vi "Powerboard_Controller Test.vi"() -> ()   [LabVIEW 2018]
uses:
  LVU examples/SubVIs/Global textParse.vi
  <instrlib>/RIGOL DS1000 Series/RIGOL DS1000 Series.lvlib
  <vilib>/measure/NI_MAPro.lvlib
  <vilib>/measure/mascope.llb/Amplitude and Levels 1 chan.vi
  <vilib>/Utility/file.llb/Read Delimited Spreadsheet (string).vi
panel:
  out "Y min 2":dbl format="%0.2f"
  out "Y max 2":dbl format="%0.2f"
  out "Y min":dbl format="%0.2f"
  out "Y max":dbl format="%0.2f"
  out "Digital Display 2":dbl
  out "Boolean 3":bool
  out "Boolean 2":bool
  out "Boolean":bool
  out "Out 5":dbl
  out "Out 4":dbl
  out "Out 3":dbl
  out "Out 2":dbl
  out "Out 1":dbl
  in  "Tab Control":T1(tab)
  in  "Department":string
  in  "Operator Name":string="ID-0"
  in  "SpecSheet Scan":string
  out "Good":bool
  in  "E-STOP":bool
  out "Bad":bool
  out "File Path":string
  out "File Name":string
  in  "Department":bool
  in  "Name":bool
  out "Boolean 4":bool
  out "Boolean 5":bool
  in  "Barcode Scan":string
  in  "VISA Waveform Generator":refnum<visa-resource-name>
  in  "VISA MultiMeter":refnum<visa-resource-name>
  in  "VISA Oscilloscope":refnum<visa-resource-name>
  out "Vmicr0":bool
  out "Vfet Driver":bool
  out "Primary":dbl(slide) caption="Secondary" scale=0.0..3000.0
  in  "Serial Port":refnum<visa-resource-name>
  out "I limit":bool
  out "I Limit":string
  out "Firmware 2":bool
  out "Firmware":string
  out "IRcomp 2":bool
  out "IRcomp":string
  out "DG":bool
  out "DM":bool
  out "DS":bool
  out "bar code read":string
  in  "stop":bool
  in  "bar code":string
  out "concatenated string":string
  out "error?":bool
  in  "Documentation":u16(ring) items=["SW Version", "Powerboard_Controller", "Equipment Test"]
  out "SW Version":string[][](array[string])
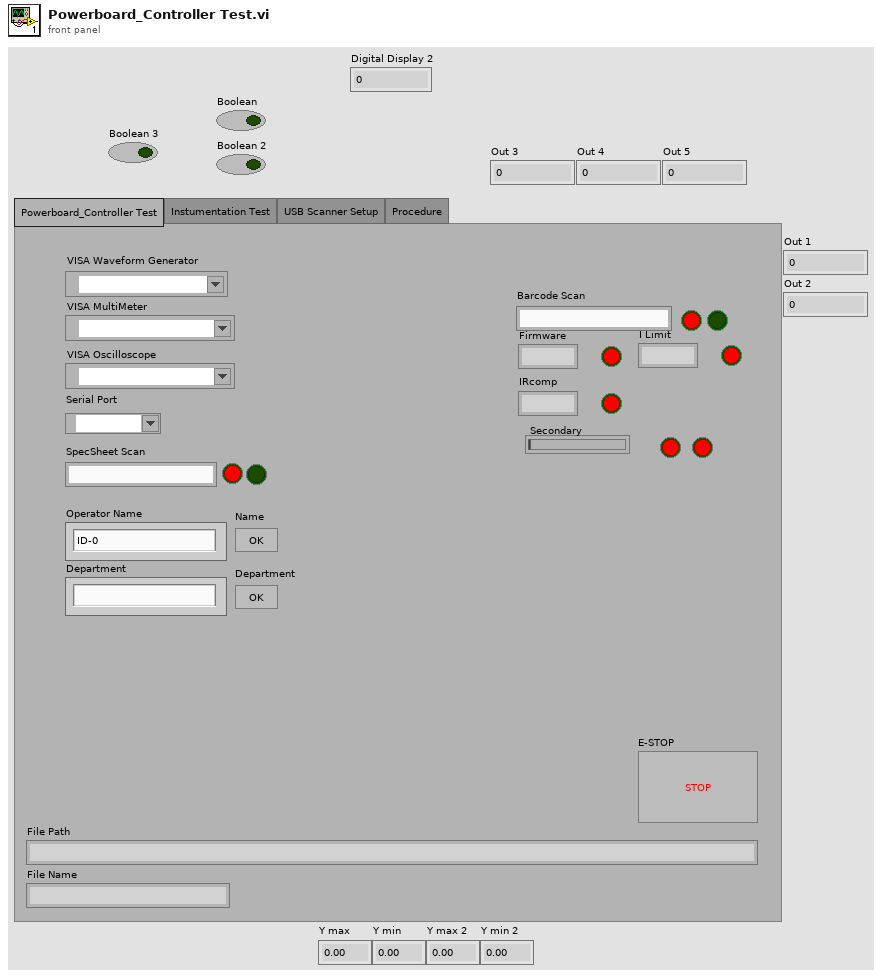
[diagram p1: front panel]
types:
  T1 = enum32{"Powerboard_Controller Test", "Instumentation Test", "USB Scanner Setup", "Procedure"}
  T2 = enum16{"Always On", "Always Off", "Off While Running"}
  T3 = enum16{"Initialize", "SW Read", "Secondary", "Incline", "Primary", "Motor", "Another", "Fail", "Close"}
  T4 = enum16{"Console unloaded", "Console loaded", "pass through", "fail"}
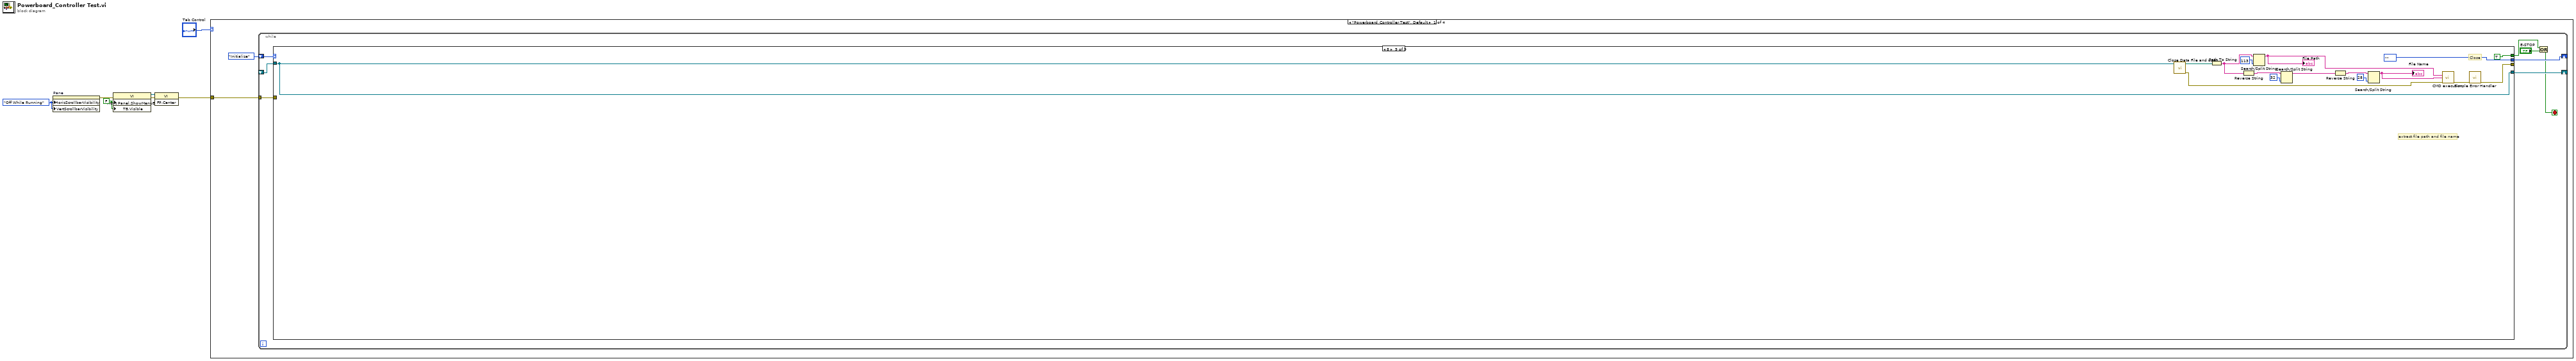
[diagram p0: block diagram]
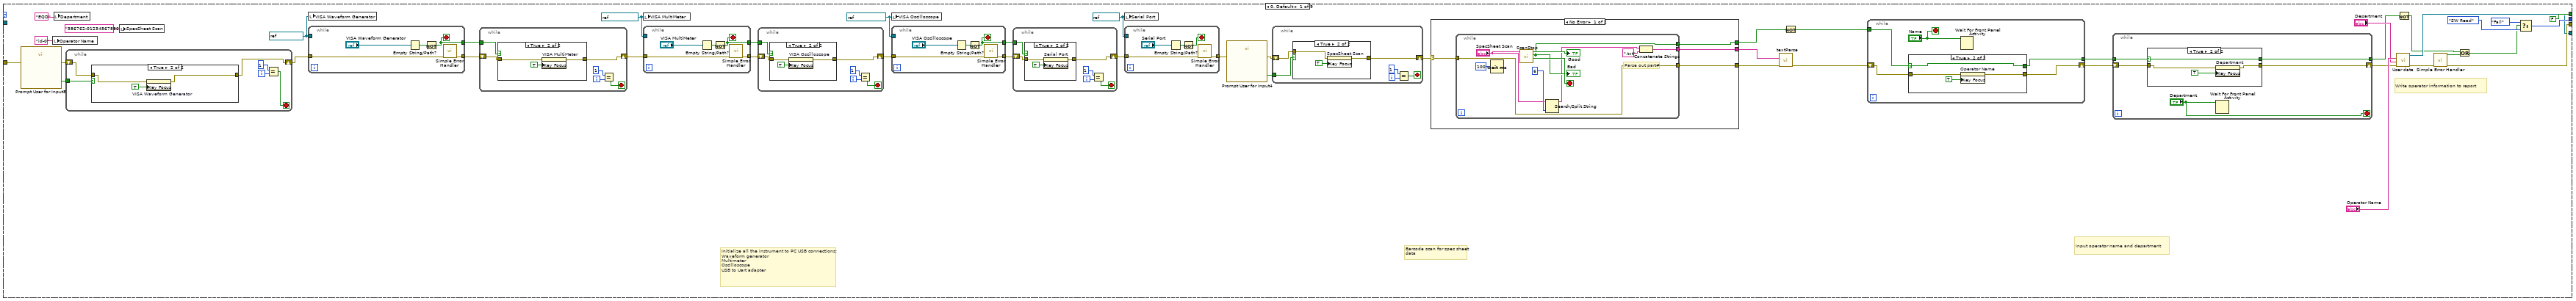
[diagram p2: hidden frame]
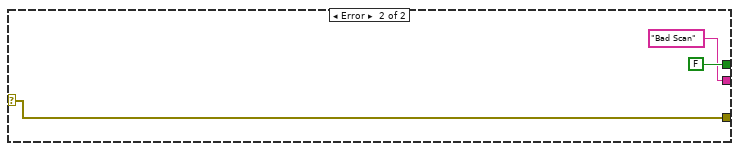
[diagram p10: hidden frame]
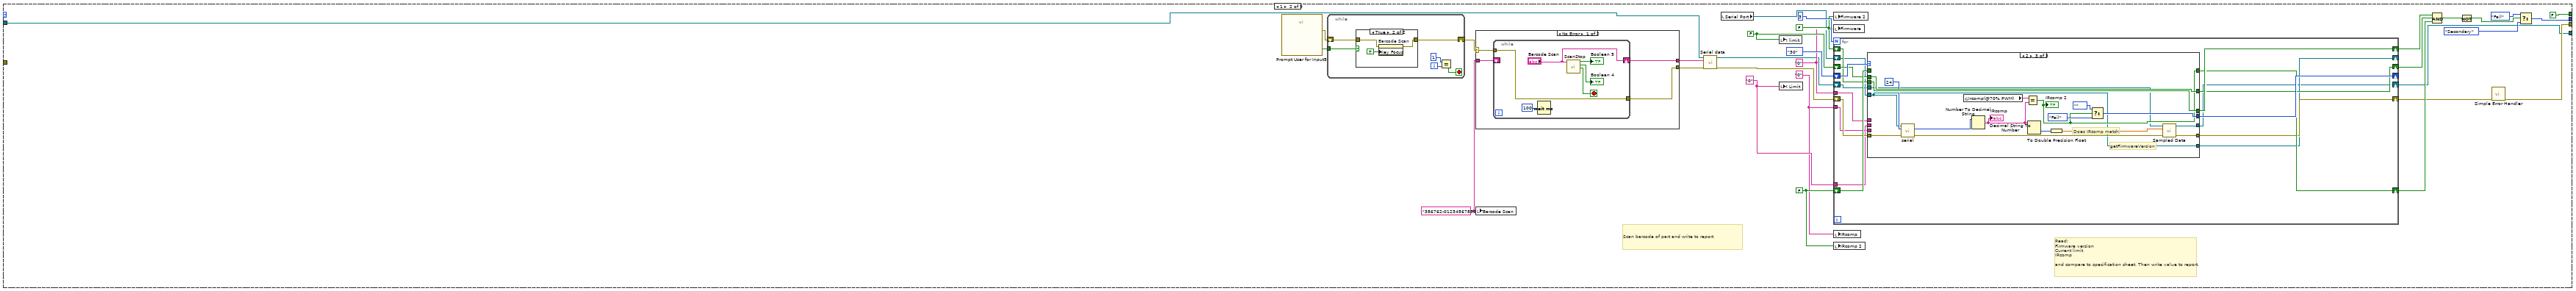
[diagram p11: hidden frame]
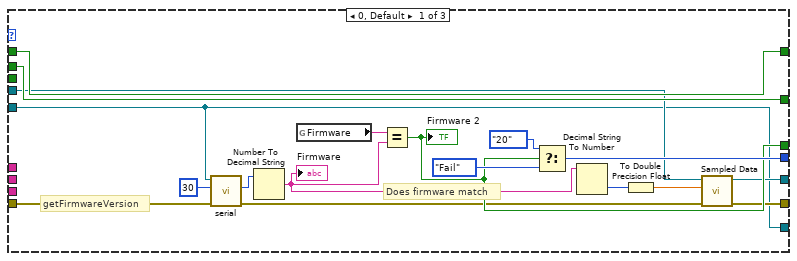
[diagram p12: hidden frame]
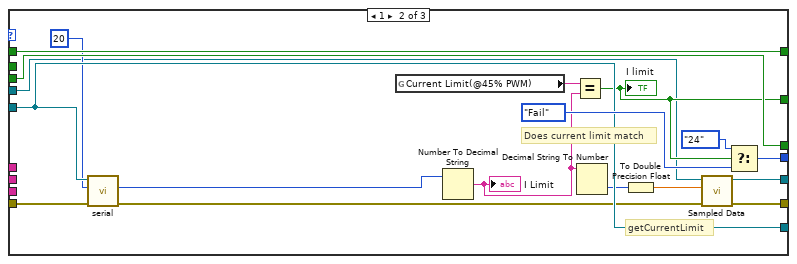
[diagram p13: hidden frame]
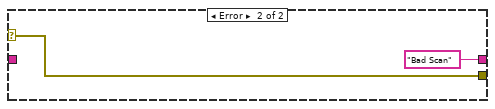
[diagram p15: hidden frame]
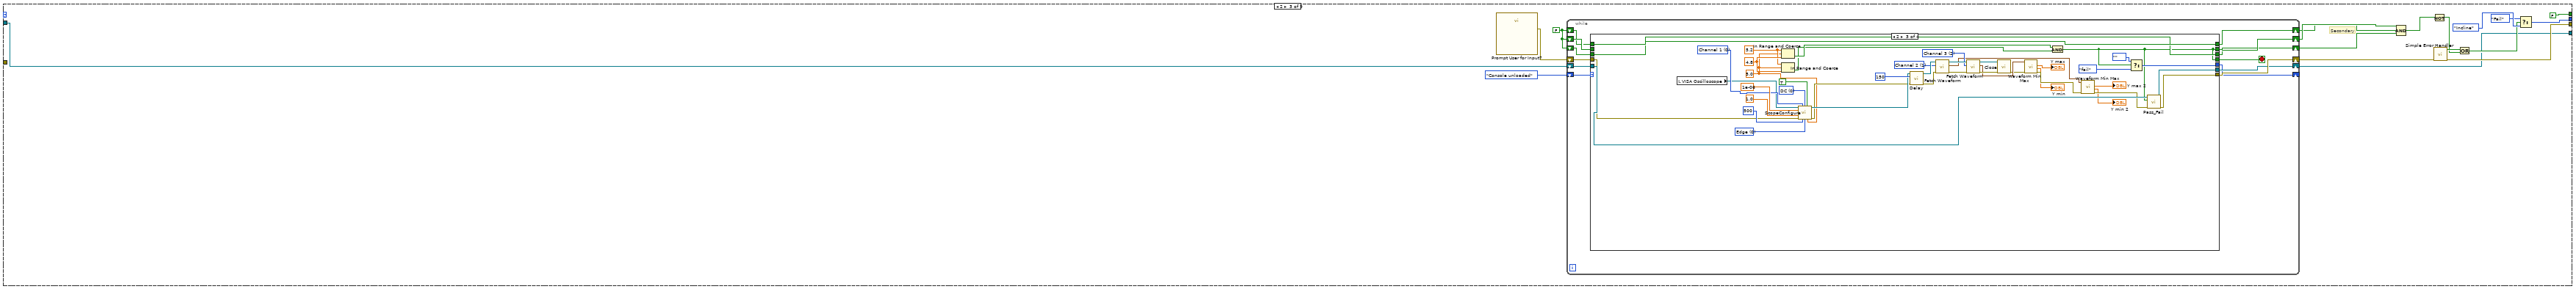
[diagram p16: hidden frame]
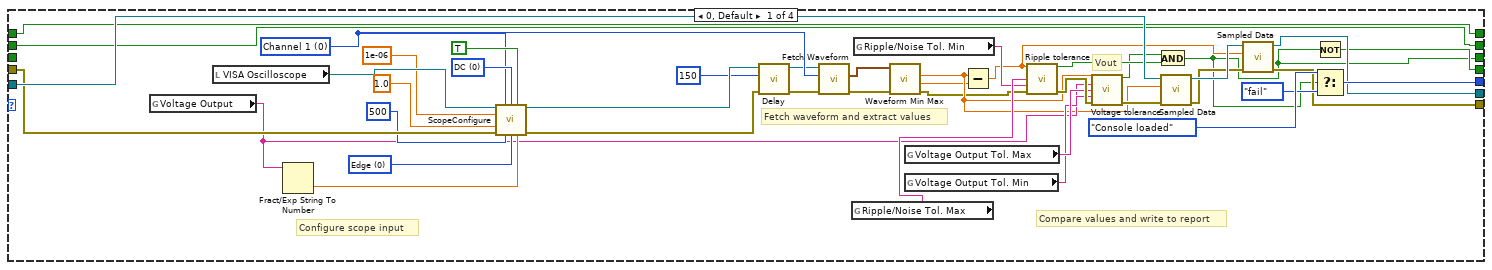
[diagram p17: hidden frame]
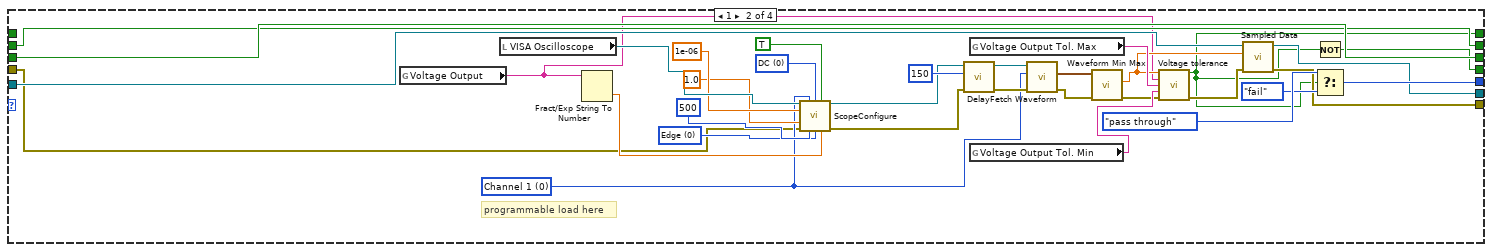
[diagram p18: hidden frame]
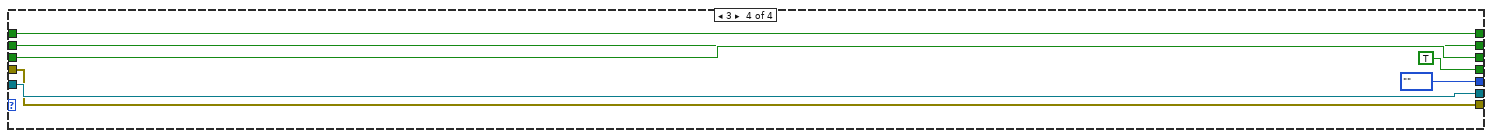
[diagram p19: hidden frame]
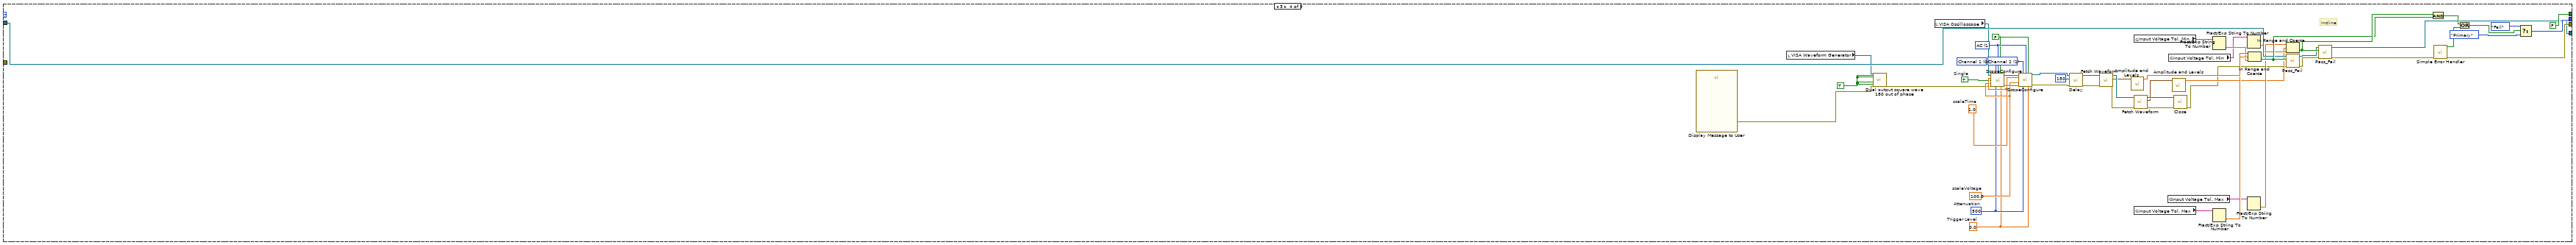
[diagram p20: hidden frame]
diagram:
  w3 = FALSE ("Front Panel Window:Show Menu Bar")
  w2 = T2."Off While Running" ("Vertical Scrollbar Visibility")
  n1 = property on="Pane" class="Pane"("HorizScrollbarVisibility"=w2, "VertScrollbarVisibility"=w2) -> (error out=w4:errorcluster)  [unwired: 2 in, 1 out]
  n2 = property class="VI"(error in=w4, "Front Panel.ShowMenuBar"=w3, "TB.Visible"=w3) -> (reference out=w6:refnum<vi>, error out=w5:errorcluster)  [unwired: 1 in]
  n3 = invoke class="VI" method="FP.Center"(reference=w6, error in=w5) -> (error out=w1:errorcluster)  [unwired: 1 in, 2 out]
  n4 = case shown="\"Powerboard_Controller Test\", Default" "Tab Control" {
    tunnel: w1 -> [w8 _ _ _]
    frame "Powerboard_Controller Test", Default {
      n5 = while {
        shift-right: [w17] -> _
        shift-left: T3."Initialize" -> [w16]
        shift-right: [w15] -> _
        shift-left: _ -> [w14]
        tunnel: w8 -> [w10]
        stop <- w11 stop-if-true
        n6 = case shown="8" w16 {
          tunnel: [w62 w200 w309 w501 w532 w583 w597 T3."Another" enum16{""}.""] -> w17
          tunnel: [w61 w201 w310 w500 w531 w584 w596 w605 w621] -> _
          tunnel: [w50 w174 w303 w491 w527 w580 w595 w603 w619] -> w15
          tunnel: w14 -> [_ w190 w304 w493 w529 w578 w595 w602 w619]
          tunnel: [FALSE ("error?") FALSE ("error?") FALSE ("error?") FALSE ("error?") FALSE ("error?") FALSE ("error?") FALSE ("error?") w604 TRUE ("error?")] -> w12
          tunnel: w10 -> [w22 _ _ _ _ _ _ _ _]
          frame 0, Default {
            w26 = refnum<visa-resource-name> "COM4" ("VISA MultiMeter")
            w25 = refnum<visa-resource-name> "DemoScope" ("VISA MultiMeter")
            w24 = refnum<visa-resource-name> "Multimeter" ("VISA MultiMeter")
            w23 = refnum<visa-resource-name> "Generator" ("VISA Waveform Generator")
            # "Write operator information to report"
            # "Input operator name and department"
            # "Barcode scan for spec sheet data"
            # "Initialize all the instrument to PC USB connections:\nWaveform generator\nMultimeter\nOscilloscope\nUSB to Uart adapter"
            n7 = call "Prompt User for Input8"("error in (no error)"=w22) -> ("OK"=w28:bool, "error out"=w27:errorcluster)  [unwired: 17 in]
            n8 = local write "Operator Name"("id-0") -> ()
            n9 = local write "Department"("EQD") -> ()
            n10 = while {
              tunnel: w28 -> [w116]
              shift-right: [w118] -> w29
              shift-left: w27 -> [w117]
              i -> [w115]
              stop <- w113 stop-if-true
              n11 = case shown="True" w116 {
                tunnel: [w119 w122] -> w118
                tunnel: w117 -> [w119 w121]
                frame False {
                }
                frame True {
                  n12 = property on="VISA Waveform Generator" class="VISAName"(error in=w121, "Key Focus"=TRUE) -> (error out=w122:errorcluster)  [unwired: 1 in, 1 out]
                }
              }
              n13 = Equal?(x=1, y=w115) -> (x = y?=w113:bool)
            }
            n14 = local write "SpecSheet Scan"("386762-01234567890") -> ()
            n15 = local write "VISA Waveform Generator"(w23) -> ()
            n16 = while {
              tunnel: w29 -> [w112]
              tunnel: [w111] -> w30
              tunnel: w23 -> [_]
              tunnel: [w108] -> w31
              stop <- w108 stop-if-true
              n17 = Empty String/Path?(string/path="VISA Waveform Generator") -> (empty?=w109:bool)
              n18 = Not(x=w109) -> (.not. x?=w108:bool)
              n19 = call <vilib>:"Simple Error Handler.vi"("error in (no error)"=w112) -> ("error out"=w111:errorcluster)  [unwired: 4 in, 4 out]
            }
            n20 = while {
              tunnel: w31 -> [w101]
              shift-right: [w103] -> w32
              shift-left: w30 -> [w102]
              i -> [w100]
              stop <- w98 stop-if-true
              n21 = case shown="True" w101 {
                tunnel: [w104 w107] -> w103
                tunnel: w102 -> [w104 w106]
                frame False {
                }
                frame True {
                  n22 = property on="VISA MultiMeter" class="VISAName"(error in=w106, "Key Focus"=TRUE) -> (error out=w107:errorcluster)  [unwired: 1 in, 1 out]
                }
              }
              n23 = Equal?(x=1, y=w100) -> (x = y?=w98:bool)
            }
            n24 = local write "VISA MultiMeter"(w24) -> ()
            n25 = while {
              tunnel: w32 -> [w97]
              tunnel: [w96] -> w34
              tunnel: [w94] -> w35
              tunnel: w24 -> [_]
              stop <- w94 stop-if-true
              n26 = Empty String/Path?(string/path="VISA MultiMeter") -> (empty?=w95:bool)
              n27 = Not(x=w95) -> (.not. x?=w94:bool)
              n28 = call <vilib>:"Simple Error Handler.vi"("error in (no error)"=w97) -> ("error out"=w96:errorcluster)  [unwired: 4 in, 4 out]
            }
            n29 = while {
              tunnel: w35 -> [w86]
              shift-right: [w88] -> w33
              shift-left: w34 -> [w87]
              i -> [w85]
              stop <- w83 stop-if-true
              n30 = case shown="True" w86 {
                tunnel: [w89 w92] -> w88
                tunnel: w87 -> [w89 w91]
                frame False {
                }
                frame True {
                  n31 = property on="VISA Oscilloscope" class="VISAName"(error in=w91, "Key Focus"=TRUE) -> (error out=w92:errorcluster)  [unwired: 1 in, 1 out]
                }
              }
              n32 = Equal?(x=1, y=w85) -> (x = y?=w83:bool)
            }
            n33 = local write "VISA Oscilloscope"(w25) -> ()
            n34 = while {
              tunnel: w33 -> [w82]
              tunnel: [w81] -> w37
              tunnel: [w79] -> w38
              tunnel: w25 -> [_]
              stop <- w79 stop-if-true
              n35 = Empty String/Path?(string/path="VISA Oscilloscope") -> (empty?=w80:bool)
              n36 = Not(x=w80) -> (.not. x?=w79:bool)
              n37 = call <vilib>:"Simple Error Handler.vi"("error in (no error)"=w82) -> ("error out"=w81:errorcluster)  [unwired: 4 in, 4 out]
            }
            n38 = while {
              shift-right: [w73] -> w36
              shift-left: w37 -> [w72]
              tunnel: w38 -> [w68]
              i -> [w71]
              stop <- w69 stop-if-true
              n39 = case shown="True" w68 {
                tunnel: [w74 w77] -> w73
                tunnel: w72 -> [w74 w76]
                frame False {
                }
                frame True {
                  n40 = property on="Serial Port" class="VISAName"(error in=w76, "Key Focus"=TRUE) -> (error out=w77:errorcluster)  [unwired: 1 in, 1 out]
                }
              }
              n41 = Equal?(x=1, y=w71) -> (x = y?=w69:bool)
            }
            n42 = local write "Serial Port"(w26) -> ()
            n43 = while {
              tunnel: w36 -> [w67]
              tunnel: [w66] -> w21
              tunnel: w26 -> [_]
              stop <- w64 stop-if-true
              n44 = Empty String/Path?(string/path="Serial Port") -> (empty?=w65:bool)
              n45 = Not(x=w65) -> (.not. x?=w64:bool)
              n46 = call <vilib>:"Simple Error Handler.vi"("error in (no error)"=w67) -> ("error out"=w66:errorcluster)  [unwired: 4 in, 4 out]
            }
            n47 = call "Prompt User for Input4"("error in (no error)"=w21) -> ("OK"=w47:bool, "error out"=w48:errorcluster)  [unwired: 17 in]
            n48 = while {
              tunnel: w47 -> [w148]
              shift-right: [w150] -> w55
              shift-left: w48 -> [w149]
              i -> [w147]
              stop <- w145 stop-if-true
              n49 = case shown="True" w148 {
                tunnel: [w151 w154] -> w150
                tunnel: w149 -> [w151 w153]
                frame False {
                }
                frame True {
                  n50 = property on="SpecSheet Scan" class="Str"(error in=w153, "Key Focus"=TRUE) -> (error out=w154:errorcluster)  [unwired: 1 in, 1 out]
                }
              }
              n51 = Equal?(x=1, y=w147) -> (x = y?=w145:bool)
            }
            n52 = case shown="No Error" w55 {
              selector: w55 -> [w158 w171]
              tunnel: [w157 w171] -> w53
              tunnel: [w156 FALSE] -> w42
              tunnel: [w155 "Bad Scan" ("bar code")] -> w54
              frame No Error {
                n53 = while {
                  tunnel: w158 -> [w167]
                  tunnel: [w167] -> w157
                  tunnel: [w164] -> w156
                  tunnel: [w160] -> w155
                  stop <- w166 stop-if-true
                  # "Parse out part#"
                  n54 = Wait (ms)(milliseconds to wait=u32 100) -> ()  [unwired: 1 out]
                  n55 = call "ScanStop.vi"("bar code scan"="SpecSheet Scan") -> ("Boolean 3"=w166:bool, "Boolean"=w164:bool, "Boolean 2"=→"Good":bool)  [unwired: 8 in]
                  "Bad" <- w164
                  n56 = Search/Split String(string="SpecSheet Scan", offset (0)=6) -> (substring before match=w163:string)  [unwired: 1 in, 2 out]
                  n57 = Concatenate Strings(w163, ".txt" ("string")) -> (w160:string)
                }
              }
              frame Error {
              }
            }
            n58 = call "textParse.vi"("error in (no error)"=w53, "file name"=w54) -> ("error out"=w46:errorcluster)  [unwired: 7 in, 2 out]
            n59 = Not(x=w42) -> (.not. x?=w39:bool)
            n60 = while {
              shift-right: [w138] -> w45
              shift-left: w46 -> [w137]
              tunnel: [w136] -> w43
              tunnel: w39 -> [w134]
              stop <- "Name" stop-if-true
              n61 = case shown="True" w134 {
                selector: w134 -> [w139 w141]
                tunnel: [w140 w142] -> w138
                tunnel: w137 -> [w140 w143]
                tunnel: [w139 w141] -> w136
                frame False {
                }
                frame True {
                  n62 = property on="Operator Name" class="Str"(error in=w143, "Key Focus"=TRUE) -> (error out=w142:errorcluster)  [unwired: 1 in, 1 out]
                }
              }
              n63 = Wait For Front Panel Activity(3:"Name") -> ()  [unwired: 2 in, 1 out]
            }
            n64 = while {
              shift-right: [w127] -> w44
              shift-left: w45 -> [w126]
              tunnel: w43 -> [w125]
              tunnel: [w124] -> w41
              stop <- "Department" stop-if-true
              n65 = case shown="True" w125 {
                selector: w125 -> [w128 w130]
                tunnel: [w129 w131] -> w127
                tunnel: w126 -> [w129 w132]
                tunnel: [w128 w130] -> w124
                frame False {
                }
                frame True {
                  n66 = property on="Department" class="Str"(error in=w132, "Key Focus"=TRUE) -> (error out=w131:errorcluster)  [unwired: 1 in, 1 out]
                }
              }
              n67 = Wait For Front Panel Activity(3:"Department") -> ()  [unwired: 2 in, 1 out]
            }
            n68 = call "User data.vi"("Error In"=w44, "Factory Name"="Department", "Operator Name"="Operator Name") -> ("error out"=w49:errorcluster, "refnum out"=w50:refnum<file>)  [unwired: 7 in]
            n69 = Not(x=w41) -> (.not. x?=w40:bool)
            n70 = call <vilib>:"Simple Error Handler.vi"("error in (no error)"=w49) -> ("error?"=w56:bool, "error out"=w61:errorcluster)  [unwired: 4 in, 3 out]
            n71 = Or(x=w40, y=w56) -> (x .or. y?=w58:bool)
            n72 = Select(t=T3."Fail", s=w58, f=T3."SW Read") -> (s? t:f=w62:T3)
          }
          frame 1 {
            w172 = "386762-01234567890"
            w176 = "0" ("IRcomp")
            w177 = "0" ("I Limit")
            w178 = "0" ("Firmware")
            w187 = FALSE ("IRcomp")
            w186 = FALSE ("I limit")
            w185 = FALSE ("Firmware")
            # "Read:\nFirmware version\nCurrent limit\nIRcomp\n\nand compare to specification sheet. Then write value to report."
            # "Scan barcode of part and write to report"
            n73 = call "Prompt User for Input5"() -> ("OK"=w191:bool, "error out"=w192:errorcluster)  [unwired: 18 in]
            n74 = while {
              tunnel: w191 -> [w276]
              shift-right: [w278] -> w195
              shift-left: w192 -> [w277]
              i -> [w275]
              stop <- w273 stop-if-true
              n75 = case shown="True" w276 {
                tunnel: [w279 w282] -> w278
                tunnel: w277 -> [w279 w281]
                frame False {
                }
                frame True {
                  n76 = property on="Barcode Scan" class="Str"(error in=w281, "Key Focus"=TRUE) -> (error out=w282:errorcluster)  [unwired: 1 in, 1 out]
                }
              }
              n77 = Equal?(x=1, y=w275) -> (x = y?=w273:bool)
            }
            n78 = case shown="No Error" w195 {
              selector: w195 -> [w285 w294]
              tunnel: [w286 "Bad Scan" ("bar code")] -> w193
              tunnel: [w284 w294] -> w194
              tunnel: w172 -> [w283 _]
              frame No Error {
                n79 = while {
                  tunnel: w285 -> [w291]
                  tunnel: [w291] -> w284
                  shift-right: ["Barcode Scan"] -> w286
                  shift-left: w283 -> [_]
                  stop <- w289 stop-if-true
                  n80 = Wait (ms)(milliseconds to wait=u32 100) -> ()  [unwired: 1 out]
                  n81 = call "ScanStop.vi"("bar code scan"="Barcode Scan") -> ("Boolean 3"=w289:bool, "Boolean"=→"Boolean 4":bool, "Boolean 2"=→"Boolean 5":bool)  [unwired: 8 in]
                }
              }
              frame Error {
              }
            }
            n82 = local write "Barcode Scan"(w172) -> ()
            n83 = call "Serial data.vi"("error in"=w194, "Serial Number"=w193, "refnum in"=w190) -> ("error out"=w181:errorcluster, "refnum out"=w175:refnum<file>)  [unwired: 7 in]
            n84 = local read "Serial Port"() -> (w173:refnum<visa-resource-name>)
            n85 = local write "I limit"(w186) -> ()
            n86 = local write "I Limit"(w177) -> ()
            n87 = local write "Firmware 2"(w185) -> ()
            n88 = local write "Firmware"(w178) -> ()
            n89 = for {
              N: 3 -> [_]
              shift-right: [w217] -> _
              shift-left: enum16{"30", "20", "24"}."30" -> [w218]
              shift-right: [w213] -> w184
              shift-left: w185 -> [w214]
              shift-right: [w212] -> w183
              shift-left: w186 -> [w215]
              shift-right: [w211] -> w182
              shift-left: w187 -> [w216]
              shift-right: [w209] -> w180
              shift-left: w181 -> [w210]
              shift-right: [w207] -> _
              shift-left: w173 -> [w208]
              tunnel: w178 -> [w206]
              tunnel: w177 -> [w205]
              tunnel: w176 -> [w204]
              shift-right: [w202] -> w174
              shift-left: w175 -> [w203]
              n90 = case shown="2" w218 {
                tunnel: [w233 w252 w270] -> w217
                tunnel: w216 -> [w230 w249 _]
                tunnel: w215 -> [w231 _ w266]
                tunnel: w214 -> [_ w250 w267]
                tunnel: [w227 w250 w267] -> w213
                tunnel: [w231 w244 w266] -> w212
                tunnel: [w230 w249 w263] -> w211
                tunnel: w210 -> [w229 w248 w265]
                tunnel: [w223 w242 w259] -> w209
                tunnel: w208 -> [w219 w247 w255]
                tunnel: [w219 w247 w255] -> w207
                tunnel: w206 -> [_ _ _]
                tunnel: w205 -> [_ _ _]
                tunnel: w204 -> [_ _ _]
                tunnel: w203 -> [w225 w241 w261]
                tunnel: [w226 w243 w262] -> w202
                frame 0, Default {
                  # "Does firmware match"
                  # "getFirmwareVersion"
                  n91 = call "serial.vi"("error in (no error)"=w229, "Numeric"=30, "Serial Port"=w219) -> ("error out"=w224:errorcluster, "Value"=w236:i8)  [unwired: 5 in]
                  n92 = Number To Decimal String(number=w236) -> (decimal integer string=w222:string)  [unwired: 1 in]
                  "Firmware" <- w222
                  n93 = global read "Global textParse.vi" "Firmware"() -> (w235:string)
                  n94 = Equal?(x=w235, y=w222) -> (x = y?=w227:bool)
                  "Firmware 2" <- w227
                  n95 = Select(t=enum16{"30", "20", "24", "Fail"}."20", s=w227, f=enum16{"30", "20", "24", "Fail"}."Fail") -> (s? t:f=w233:enum16{"30", "20", "24", "Fail"})
                  n96 = Decimal String To Number(string=w222) -> (number=w221:i32)  [unwired: 2 in, 1 out]
                  n97 = To Double Precision Float(number=w221) -> (double precision float=w220:dbl)
                  n98 = call "Sampled Data.vi"("Error In"=w224, "Data Sample"=w220, "refnum in"=w225) -> ("error out"=w223:errorcluster, "refnum out"=w226:refnum<file>)  [unwired: 7 in]
                }
                frame 1 {
                  # "Does current limit match"
                  # "getCurrentLimit"
                  n99 = call "serial.vi"("error in (no error)"=w248, "Numeric"=20, "Serial Port"=w247) -> ("error out"=w240:errorcluster, "Value"=w254:i8)  [unwired: 5 in]
                  n100 = global read "Global textParse.vi" "Current Limit(@45% PWM)"() -> (w245:string)
                  n101 = Number To Decimal String(number=w254) -> (decimal integer string=w239:string)  [unwired: 1 in]
                  "I Limit" <- w239
                  n102 = Equal?(x=w245, y=w239) -> (x = y?=w244:bool)
                  "I limit" <- w244
                  n103 = Decimal String To Number(string=w239) -> (number=w238:i32)  [unwired: 2 in, 1 out]
                  n104 = To Double Precision Float(number=w238) -> (double precision float=w237:dbl)
                  n105 = call "Sampled Data.vi"("Error In"=w240, "Data Sample"=w237, "refnum in"=w241) -> ("error out"=w242:errorcluster, "refnum out"=w243:refnum<file>)  [unwired: 7 in]
                  n106 = Select(t=enum16{"30", "20", "24", "Fail"}."24", s=w244, f=enum16{"30", "20", "24", "Fail"}."Fail") -> (s? t:f=w252:enum16{"30", "20", "24", "Fail"})
                }
                frame 2 {
                  # "Does IRcomp match"
                  # "getFirmwareVersion"
                  n107 = call "serial.vi"("error in (no error)"=w265, "Numeric"=24, "Serial Port"=w255) -> ("error out"=w260:errorcluster, "Value"=w272:i8)  [unwired: 5 in]
                  n108 = global read "Global textParse.vi" "Ircomp(@70% PWM)"() -> (w271:string)
                  n109 = Number To Decimal String(number=w272) -> (decimal integer string=w258:string)  [unwired: 1 in]
                  "IRcomp" <- w258
                  n110 = Equal?(x=w271, y=w258) -> (x = y?=w263:bool)
                  "IRcomp 2" <- w263
                  n111 = Decimal String To Number(string=w258) -> (number=w257:i32)  [unwired: 2 in, 1 out]
                  n112 = To Double Precision Float(number=w257) -> (double precision float=w256:dbl)
                  n113 = Select(t=enum16{""}."", s=w263, f=enum16{"30", "20", "24", "Fail"}."Fail") -> (s? t:f=w270:u16)
                  n114 = call "Sampled Data.vi"("Error In"=w260, "Data Sample"=w256, "refnum in"=w261) -> ("error out"=w259:errorcluster, "refnum out"=w262:refnum<file>)  [unwired: 7 in]
                }
              }
            }
            n115 = local write "IRcomp"(w176) -> ()
            n116 = local write "IRcomp 2"(w187) -> ()
            n117 = Compound Arithmetic op=AND(w184, w183, w182) -> (w179:bool)
            n118 = Not(x=w179) -> (.not. x?=w197:bool)
            n119 = call <vilib>:"Simple Error Handler.vi"("error in (no error)"=w180) -> ("error out"=w201:errorcluster)  [unwired: 4 in, 4 out]
            n120 = Select(t=T3."Fail", s=w197, f=T3."Secondary") -> (s? t:f=w200:T3)
          }
          frame 2 {
            w296 = FALSE
            # "Secondary"
            n121 = call "Prompt User for Input7"() -> ("error out"=w302:errorcluster)  [unwired: 18 in, 1 out]
            n122 = while {
              shift-right: [w324] -> w305
              shift-left: w302 -> [w323]
              shift-right: [w314] -> w298
              shift-left: w296 -> [w322]
              shift-right: [w321] -> w303
              shift-left: w304 -> [w320]
              shift-right: [w319] -> _
              shift-left: T4."Console unloaded" -> [w325]
              shift-right: [w315] -> w299
              shift-left: w296 -> [w317]
              shift-right: [w316] -> w300
              shift-left: w296 -> [w318]
              stop <- w313 stop-if-true
              n123 = case shown="2" w325 {
                tunnel: [w367 w396 w419 enum16{""}.""] -> w319
                tunnel: [w348 w390 w430 w450] -> w314
                tunnel: [w362 w393 w435 w446] -> w324
                tunnel: w323 -> [w344 w369 w402 w446]
                tunnel: [w361 w392 w436 w447] -> w321
                tunnel: w322 -> [_ w390 w430 w450]
                tunnel: w320 -> [w360 w391 w434 w447]
                tunnel: [w350 w382 w431 w449] -> w315
                tunnel: [w351 w389 w413 w448] -> w316
                tunnel: w318 -> [w351 w389 _ w448]
                tunnel: w317 -> [w350 _ w431 w449]
                tunnel: [w349 w383 w413 TRUE] -> w313
                frame 0, Default {
                  w332 = u16 0 items=["Edge", "Pulse", "Video", "Pattern", "Duration"] ("Trigger Type (0: Edge)")
                  w340 = u16 0 items=["DC", "AC", "Ground"] ("Vertical Coupling (0: DC)")
                  w338 = u16 0 items=["Channel 1", "Channel 2", "Channel 3", "Channel 4"] ("Channel (0: Channel 1)")
                  # "Compare values and write to report"
                  # "Fetch waveform and extract values"
                  # "Configure scope input"
                  # "Vout"
                  n124 = global read "Global textParse.vi" "Voltage Output"() -> (w330:string)
                  n125 = local read "VISA Oscilloscope"() -> (w346:refnum<visa-resource-name>)
                  n126 = Fract/Exp String To Number(string=w330) -> (number=w331:dbl)  [unwired: 3 in, 1 out]
                  n127 = call "ScopeConfigure.vi"("VISA resource name"=w346, "Channel (0: Channel 1)"=w338, "Vertical Coupling (0: DC)"=w340, "BW Selector"=TRUE, "scaleTime"=1e-06, "scaleVoltage"=1.0, "error in (no error)"=w344, "Attenuation"=500, "Trigger Type (0: Edge)"=w332, "Trigger Level"=w331) -> ("VISA resource name out"=w335:refnum<visa-resource-name>, "error out"=w347:errorcluster)  [unwired: 4 in]
                  n128 = call <instrlib>:"Delay.vi"("error in (no error)"=w347, "Delay (ms)"=u32 150, "VISA resource name"=w335) -> ("error out"=w337:errorcluster, "VISA resource name out"=w336:refnum<visa-resource-name>)  [unwired: 7 in]
                  n129 = call <instrlib>:"Fetch Waveform.vi"("error in (no error)"=w337, "Channel (0: Channel 1)"=w338, "VISA resource name"=w336) -> ("error out"=w333:errorcluster, "Waveform Data"=w339:waveform(dbl))  [unwired: 6 in, 1 out]
                  n130 = global read "Global textParse.vi" "Ripple/Noise Tol. Max"() -> (w359:string)
                  n131 = global read "Global textParse.vi" "Ripple/Noise Tol. Min"() -> (w358:string)
                  n132 = call <vilib>:"Waveform Min Max.vi"("error in (no error)"=w333, "waveform in"=w339) -> ("error out"=w327:errorcluster, "Y min"=w328:dbl, "Y max"=w329:dbl)  [unwired: 4 in, 3 out]
                  n133 = global read "Global textParse.vi" "Voltage Output Tol. Max"() -> (w355:string)
                  n134 = global read "Global textParse.vi" "Voltage Output Tol. Min"() -> (w354:string)
                  n135 = Subtract(x=w329, y=w328) -> (x-y=w326:dbl)
                  n136 = call "Ripple tolerance.vi"("Data Sample"=w326, "Upper"=w359, "Lower"=w358, "error in (no error)"=w327) -> ("Boolean"=w353:bool, "error out"=w357:errorcluster)  [unwired: 10 in]
                  n137 = call "Voltage tolerance.vi"("Data Sample"=w329, "Spec Output"=w330, "Upper"=w355, "Lower"=w354, "error in (no error)"=w357) -> ("Boolean"=w352:bool, "error out"=w356:errorcluster)  [unwired: 9 in]
                  n138 = And(x=w352, y=w353) -> (x .and. y?=w348:bool)
                  n139 = call "Sampled Data.vi"("Error In"=w356, "Data Sample"=w329, "refnum in"=w360) -> ("error out"=w363:errorcluster, "refnum out"=w364:refnum<file>)  [unwired: 7 in]
                  n140 = call "Sampled Data.vi"("Error In"=w363, "Data Sample"=w326, "refnum in"=w364) -> ("error out"=w362:errorcluster, "refnum out"=w361:refnum<file>)  [unwired: 7 in]
                  n141 = Not(x=w348) -> (.not. x?=w349:bool)
                  n142 = Select(t=T4."Console loaded", s=w348, f=T4."fail") -> (s? t:f=w367:T4)
                }
                frame 1 {
                  w373 = u16 0 items=["Edge", "Pulse", "Video", "Pattern", "Duration"] ("Trigger Type (0: Edge)")
                  w378 = u16 0 items=["DC", "AC", "Ground"] ("Vertical Coupling (0: DC)")
                  w370 = u16 0 items=["Channel 1", "Channel 2", "Channel 3", "Channel 4"] ("Channel (0: Channel 1)")
                  # "programmable load here"
                  n143 = global read "Global textParse.vi" "Voltage Output"() -> (w368:string)
                  n144 = local read "VISA Oscilloscope"() -> (w379:refnum<visa-resource-name>)
                  n145 = Fract/Exp String To Number(string=w368) -> (number=w380:dbl)  [unwired: 3 in, 1 out]
                  n146 = call "ScopeConfigure.vi"("VISA resource name"=w379, "Channel (0: Channel 1)"=w370, "Vertical Coupling (0: DC)"=w378, "BW Selector"=TRUE, "scaleTime"=1e-06, "scaleVoltage"=1.0, "error in (no error)"=w369, "Attenuation"=500, "Trigger Type (0: Edge)"=w373, "Trigger Level"=w380) -> ("VISA resource name out"=w372:refnum<visa-resource-name>, "error out"=w371:errorcluster)  [unwired: 4 in]
                  n147 = call <instrlib>:"Delay.vi"("error in (no error)"=w371, "Delay (ms)"=u32 150, "VISA resource name"=w372) -> ("error out"=w400:errorcluster, "VISA resource name out"=w399:refnum<visa-resource-name>)  [unwired: 7 in]
                  n148 = global read "Global textParse.vi" "Voltage Output Tol. Max"() -> (w388:string)
                  n149 = global read "Global textParse.vi" "Voltage Output Tol. Min"() -> (w387:string)
                  n150 = call <instrlib>:"Fetch Waveform.vi"("error in (no error)"=w400, "Channel (0: Channel 1)"=w370, "VISA resource name"=w399) -> ("error out"=w398:errorcluster, "Waveform Data"=w397:waveform(dbl))  [unwired: 6 in, 1 out]
                  n151 = call <vilib>:"Waveform Min Max.vi"("error in (no error)"=w398, "waveform in"=w397) -> ("error out"=w385:errorcluster, "Y max"=w386:dbl)  [unwired: 4 in, 4 out]
                  n152 = call "Voltage tolerance.vi"("Data Sample"=w386, "Spec Output"=w368, "Upper"=w388, "Lower"=w387, "error in (no error)"=w385) -> ("Boolean"=w382:bool, "error out"=w384:errorcluster)  [unwired: 9 in]
                  n153 = call "Sampled Data.vi"("Error In"=w384, "Data Sample"=w386, "refnum in"=w391) -> ("error out"=w393:errorcluster, "refnum out"=w392:refnum<file>)  [unwired: 7 in]
                  n154 = Not(x=w382) -> (.not. x?=w383:bool)
                  n155 = Select(t=T4."pass through", s=w382, f=T4."fail") -> (s? t:f=w396:T4)
                }
                frame 2 {
                  w406 = u16 0 items=["Edge", "Pulse", "Video", "Pattern", "Duration"] ("Trigger Type (0: Edge)")
                  w408 = u16 0 items=["DC", "AC", "Ground"] ("Vertical Coupling (0: DC)")
                  w407 = u16 0 items=["Channel 1", "Channel 2", "Channel 3", "Channel 4"] ("Channel (0: Channel 1)")
                  w401 = 5.0
                  w426 = u16 2 items=["Channel 1", "Channel 2", "Channel 3", "Channel 4"] ("Channel (0: Channel 1)")
                  w433 = 4.8 ("lower limit")
                  w432 = 5.2 ("upper limit")
                  w441 = u16 1 items=["Channel 1", "Channel 2", "Channel 3", "Channel 4"] ("Channel (0: Channel 1)")
                  n156 = local read "VISA Oscilloscope"() -> (w405:refnum<visa-resource-name>)
                  n157 = In Range and Coerce(upper limit=w432, x=w401, lower limit=w433) -> (In Range?=w438:bool)  [unwired: 1 out]
                  n158 = In Range and Coerce(upper limit=w432, x=w401, lower limit=w433) -> (In Range?=w437:bool)  [unwired: 1 out]
                  n159 = call "ScopeConfigure.vi"("VISA resource name"=w405, "Channel (0: Channel 1)"=w407, "Vertical Coupling (0: DC)"=w408, "BW Selector"=TRUE, "scaleTime"=1e-06, "scaleVoltage"=1.0, "error in (no error)"=w402, "Attenuation"=500, "Trigger Type (0: Edge)"=w406, "Trigger Level"=w401) -> ("VISA resource name out"=w404:refnum<visa-resource-name>, "error out"=w403:errorcluster)  [unwired: 4 in]
                  n160 = call <instrlib>:"Delay.vi"("error in (no error)"=w403, "Delay (ms)"=u32 150, "VISA resource name"=w404) -> ("error out"=w443:errorcluster, "VISA resource name out"=w442:refnum<visa-resource-name>)  [unwired: 7 in]
                  n161 = call <instrlib>:"Fetch Waveform.vi"("error in (no error)"=w443, "Channel (0: Channel 1)"=w441, "VISA resource name"=w442) -> ("error out"=w439:errorcluster, "Waveform Data"=w424:waveform(dbl), "VISA resource name out"=w428:refnum<visa-resource-name>)  [unwired: 6 in]
                  n162 = call <instrlib>:"Fetch Waveform.vi"("error in (no error)"=w439, "Channel (0: Channel 1)"=w426, "VISA resource name"=w428) -> ("error out"=w429:errorcluster, "Waveform Data"=w425:waveform(dbl), "VISA resource name out"=w427:refnum<visa-resource-name>)  [unwired: 6 in]
                  n163 = call <instrlib>:"Close.vi"("error in (no error)"=w429, "VISA resource name"=w427) -> ("error out"=w422:errorcluster)  [unwired: 9 in]
                  n164 = call <vilib>:"Waveform Min Max.vi"("error in (no error)"=w422, "waveform in"=w425) -> ("error out"=w423:errorcluster, "Y min"=→"Y min":dbl, "Y max"=→"Y max":dbl)  [unwired: 4 in, 3 out]
                  n165 = And(x=w438, y=w437) -> (x .and. y?=w413:bool)
                  n166 = call <vilib>:"Waveform Min Max.vi"("error in (no error)"=w423, "waveform in"=w424) -> ("error out"=w421:errorcluster, "Y min"=→"Y min 2":dbl, "Y max"=→"Y max 2":dbl)  [unwired: 4 in, 3 out]
                  n167 = Select(t=enum16{""}."", s=w413, f=T4."fail") -> (s? t:f=w419:u16)
                  n168 = call "Pass_Fail.vi"("error in (no error)"=w421, "OK"=w413, "Byte Stream File in"=w434) -> ("error out"=w435:errorcluster, "Byte Stream File out"=w436:refnum<file>)  [unwired: 7 in]
                }
                frame 3 {
                }
              }
            }
            n169 = Compound Arithmetic op=AND(w300, w299, w298) -> (w297:bool)
            n170 = Not(x=w297) -> (.not. x?=w301:bool)
            n171 = call <vilib>:"Simple Error Handler.vi"("error in (no error)"=w305) -> ("error?"=w306:bool, "error out"=w310:errorcluster)  [unwired: 4 in, 3 out]
            n172 = Or(x=w306, y=w301) -> (x .or. y?=w307:bool)
            n173 = Select(t=T3."Fail", s=w307, f=T3."Incline") -> (s? t:f=w309:T3)
          }
          frame 3 {
            w452 = TRUE  # Single
            w456 = 0.0  # Trigger Level
            w457 = 500  # Attenuation
            w458 = 100.0  # scaleVoltage
            w459 = 1.0  # scaleTime
            w460 = FALSE ("BW Selector")
            w461 = u16 1 items=["DC", "AC", "Ground"] ("Vertical Coupling (0: DC)")
            w462 = u16 1 items=["Channel 1", "Channel 2", "Channel 3", "Channel 4"] ("Channel (0: Channel 1)")
            w463 = u16 0 items=["Channel 1", "Channel 2", "Channel 3", "Channel 4"] ("Channel (0: Channel 1)")
            w451 = TRUE ("Enable Output 1")
            # "Incline"
            n174 = call "Display Message to User"() -> ("error out"=w467:errorcluster)  [unwired: 10 in, 1 out]
            n175 = local read "VISA Waveform Generator"() -> (w464:refnum<visa-resource-name>)
            n176 = call "Dual output square wave 180 out of phase.vi"("VISA resource name"=w464, "Enable Output 1"=w451, "Enable Align (F: Disable) 1"=w451, "Enable Output 2"=w451, "Enable Align (F: Disable) 2"=w451, "error in (no error)"=w467) -> ("error out"=w453:errorcluster)  [unwired: 20 in, 1 out]
            n177 = local read "VISA Oscilloscope"() -> (w468:refnum<visa-resource-name>)
            n178 = call "ScopeConfigure.vi"("VISA resource name"=w468, "Channel (0: Channel 1)"=w463, "Vertical Coupling (0: DC)"=w461, "BW Selector"=w460, "scaleTime"=w459, "Single"=w452, "scaleVoltage"=w458, "error in (no error)"=w453, "Attenuation"=w457, "Trigger Level"=w456) -> ("VISA resource name out"=w466:refnum<visa-resource-name>, "error out"=w465:errorcluster)  [unwired: 4 in]
            n179 = call "ScopeConfigure.vi"("VISA resource name"=w466, "Channel (0: Channel 1)"=w462, "Vertical Coupling (0: DC)"=w461, "BW Selector"=w460, "scaleTime"=w459, "scaleVoltage"=w458, "error in (no error)"=w465, "Attenuation"=w457, "Trigger Level"=w456) -> ("VISA resource name out"=w454:refnum<visa-resource-name>, "error out"=w455:errorcluster)  [unwired: 5 in]
            n180 = call <instrlib>:"Delay.vi"("error in (no error)"=w455, "Delay (ms)"=u32 150, "VISA resource name"=w454) -> ("error out"=w477:errorcluster, "VISA resource name out"=w476:refnum<visa-resource-name>)  [unwired: 7 in]
            n181 = call <instrlib>:"Fetch Waveform.vi"("error in (no error)"=w477, "VISA resource name"=w476) -> ("error out"=w475:errorcluster, "Waveform Data"=w471:waveform(dbl), "VISA resource name out"=w474:refnum<visa-resource-name>)  [unwired: 7 in]
            n182 = call-poly <vilib>:"Amplitude and Levels.vi"("signal in"=w471) -> ("amplitude"=w490:dbl)  [unwired: 7 in, 3 out]
            n183 = call <instrlib>:"Fetch Waveform.vi"("error in (no error)"=w475, "VISA resource name"=w474) -> ("error out"=w473:errorcluster, "Waveform Data"=w470:waveform(dbl), "VISA resource name out"=w472:refnum<visa-resource-name>)  [unwired: 7 in]
            n184 = global read "Global textParse.vi" "Input Voltage Tol. Min"() -> (w489:string)
            n185 = global read "Global textParse.vi" "Input Voltage Tol. Max"() -> (w481:string)
            n186 = global read "Global textParse.vi" "Input Voltage Tol. Max"() -> (w482:string)
            n187 = global read "Global textParse.vi" "Input Voltage Tol. Min"() -> (w484:string)
            n188 = call-poly <vilib>:"Amplitude and Levels.vi"("signal in"=w470) -> ("amplitude"=w483:dbl)  [unwired: 7 in, 3 out]
            n189 = call <instrlib>:"Close.vi"("error in (no error)"=w473, "VISA resource name"=w472) -> ("error out"=w478:errorcluster)  [unwired: 9 in]
            n190 = Fract/Exp String To Number(string=w489) -> (number=w487:dbl)  [unwired: 3 in, 1 out]
            n191 = Fract/Exp String To Number(string=w481) -> (number=w488:dbl)  [unwired: 3 in, 1 out]
            n192 = Fract/Exp String To Number(string=w484) -> (number=w486:dbl)  [unwired: 3 in, 1 out]
            n193 = Fract/Exp String To Number(string=w482) -> (number=w485:dbl)  [unwired: 3 in, 1 out]
            n194 = In Range and Coerce(upper limit=w488, x=w490, lower limit=w487) -> (In Range?=w495:bool)  [unwired: 1 out]
            n195 = In Range and Coerce(upper limit=w485, x=w483, lower limit=w486) -> (In Range?=w496:bool)  [unwired: 1 out]
            n196 = call "Pass_Fail.vi"("error in (no error)"=w478, "OK"=w495, "Byte Stream File in"=w493) -> ("error out"=w479:errorcluster, "Byte Stream File out"=w480:refnum<file>)  [unwired: 7 in]
            n197 = call "Pass_Fail.vi"("error in (no error)"=w479, "OK"=w496, "Byte Stream File in"=w480) -> ("error out"=w492:errorcluster, "Byte Stream File out"=w491:refnum<file>)  [unwired: 7 in]
            n198 = And(x=w496, y=w495) -> (x .and. y?=w494:bool)
            n199 = call <vilib>:"Simple Error Handler.vi"("error in (no error)"=w492) -> ("error?"=w497:bool, "error out"=w500:errorcluster)  [unwired: 4 in, 3 out]
            n200 = Or(x=w494, y=w497) -> (x .or. y?=w498:bool)
            n201 = Select(t=T3."Fail", s=w498, f=T3."Primary") -> (s? t:f=w501:T3)
          }
          frame 4 {
            (unwired) u16 6 items=["Voltage Vpp", "Voltage Max", "Voltage Min", "Amplitude", "Voltage TOP", "Voltage Base", "Voltage Average", "Voltage RMS", "Overshoot", "Preshoot", "Frequency", "Rise Time", "Fall Time", "Period", "Positive Width", "Negative Width", "Positive Duty", "Negative Duty"] ("Measurement 2")
            (unwired) u16 6 items=["Voltage Vpp", "Voltage Max", "Voltage Min", "Amplitude", "Voltage TOP", "Voltage Base", "Voltage Average", "Voltage RMS", "Overshoot", "Preshoot", "Frequency", "Rise Time", "Fall Time", "Period", "Positive Width", "Negative Width", "Positive Duty", "Negative Duty"] ("Measurement 1")
            (unwired) u16 1 items=["Channel 1", "Channel 2", "Channel 3", "Channel 4"] ("Channel (0: Channel 1) 2")
            (unwired) u16 0 items=["Channel 1", "Channel 2", "Channel 3", "Channel 4"] ("Channel (0: Channel 1) 1")
            # "Primary"
            n202 = call "Prompt User for Input3"() -> ()  [unwired: 18 in, 2 out]
            n203 = local write "Primary"(0.0 ("Primary")) -> ()
            n204 = for {
              N: 3000 -> [_]
              i -> [w536]
              n205 = Wait (ms)(milliseconds to wait=u32 1) -> ()  [unwired: 1 out]
              n206 = To Double Precision Float(number=w536) -> (double precision float=→"Primary":dbl)
            }
            n207 = Random Number (0-1)() -> (number: 0 to 1=w522:dbl)
            n208 = global read "Global textParse.vi" "Voltage Micro Tol. Max"() -> (w505:string)
            n209 = global read "Global textParse.vi" "Voltage Micro Tol. Min"() -> (w504:string)
            n210 = Divide(x=w522, y=2.0) -> (x/y=w517:dbl)
            n211 = global read "Global textParse.vi" "Voltage Micro"() -> (w506:string)
            n212 = Add(x=w517, y=5.0) -> (x+y=w519:dbl)
            n213 = call "Voltage tolerance.vi"("Data Sample"=w519, "Spec Output"=w506, "Upper"=w505, "Lower"=w504) -> ("Boolean"=w514:bool, "error out"=w525:errorcluster)  [unwired: 10 in]
            "Vmicr0" <- w514
            n214 = global read "Global textParse.vi" "Voltage FET Driver Tol. Max"() -> (w508:string)
            n215 = global read "Global textParse.vi" "Voltage FET Driver Tol. Min"() -> (w507:string)
            n216 = global read "Global textParse.vi" "Voltage FET Driver"() -> (w509:string)
            n217 = call "Sampled Data.vi"("Error In"=w525, "Data Sample"=w519, "refnum in"=w529) -> ("error out"=w523:errorcluster, "refnum out"=w528:refnum<file>)  [unwired: 7 in]
            n218 = Add(x=w517, y=15.0) -> (x+y=w518:dbl)
            n219 = call "Voltage tolerance.vi"("Data Sample"=w518, "Spec Output"=w509, "Upper"=w508, "Lower"=w507, "error in (no error)"=w523) -> ("Boolean"=w515:bool, "error out"=w524:errorcluster)  [unwired: 9 in]
            "Vfet Driver" <- w515
            n220 = And(x=w515, y=w514) -> (x .and. y?=w513:bool)
            n221 = call "Sampled Data.vi"("Error In"=w524, "Data Sample"=w518, "refnum in"=w528) -> ("error out"=w526:errorcluster, "refnum out"=w527:refnum<file>)  [unwired: 7 in]
            n222 = Not(x=w513) -> (.not. x?=w512:bool)
            n223 = call <vilib>:"Simple Error Handler.vi"("error in (no error)"=w526) -> ("error out"=w531:errorcluster)  [unwired: 4 in, 4 out]
            n224 = Select(t=T3."Fail", s=w512, f=T3."Motor") -> (s? t:f=w532:T3)
          }
          frame 5 {
            (unwired) u16 1 items=["Channel 1", "Channel 2", "Channel 3", "Channel 4"] ("Channel (0: Channel 1) 2")
            (unwired) u16 1 items=["Channel 1", "Channel 2", "Channel 3", "Channel 4"] ("Channel (0: Channel 1) 1")
            (unwired) u16 0 items=["Channel 1", "Channel 2", "Channel 3", "Channel 4"] ("Channel (0: Channel 1) 1")
            (unwired) u16 16 items=["Voltage Vpp", "Voltage Max", "Voltage Min", "Amplitude", "Voltage TOP", "Voltage Base", "Voltage Average", "Voltage RMS", "Overshoot", "Preshoot", "Frequency", "Rise Time", "Fall Time", "Period", "Positive Width", "Negative Width", "Positive Duty", "Negative Duty"] ("Measurement 3")
            (unwired) u16 13 items=["Voltage Vpp", "Voltage Max", "Voltage Min", "Amplitude", "Voltage TOP", "Voltage Base", "Voltage Average", "Voltage RMS", "Overshoot", "Preshoot", "Frequency", "Rise Time", "Fall Time", "Period", "Positive Width", "Negative Width", "Positive Duty", "Negative Duty"] ("Measurement 2")
            (unwired) u16 1 items=["Voltage Vpp", "Voltage Max", "Voltage Min", "Amplitude", "Voltage TOP", "Voltage Base", "Voltage Average", "Voltage RMS", "Overshoot", "Preshoot", "Frequency", "Rise Time", "Fall Time", "Period", "Positive Width", "Negative Width", "Positive Duty", "Negative Duty"] ("Measurement 1")
            w560 = u16 0 items=["DC Volts", "AC Volts", "DC Current", "AC Current", "2-Wire Resistance", "4-Wire Resistance"] ("Function (0: DC Volts) 2")
            w579 = FALSE ("s")
            # "HV Bus"
            # "Motor"
            n225 = call "Prompt User for Input6"() -> ()  [unwired: 18 in, 2 out]
            n226 = local read "VISA MultiMeter"() -> (w561:refnum<visa-resource-name>)
            n227 = local read "VISA Waveform Generator"() -> (w559:refnum<visa-resource-name>)
            n228 = global read "Global textParse.vi" "Speed Pot Voltage High(@85% PWM)"() -> (w551:string)
            n229 = global read "Global textParse.vi" "Speed Pot Voltage Low(@85% PWM)"() -> (w555:string)
            n230 = global read "Global textParse.vi" "Speed Pot Voltage Mid(@85% PWM)"() -> (w542:string)
            n231 = call "Voltage measurment on multimeter.vi"("Function (0: DC Volts) 2"=w560, "VISA resource name 3"=w561) -> ("error out"=w544:errorcluster, "Digital Display"=→"Digital Display 2":dbl)  [unwired: 8 in]
            n232 = global read "Global textParse.vi" "Speed Pot Voltage Tol. Max"() -> (w554:string)
            n233 = global read "Global textParse.vi" "Speed Pot Voltage Tol. Max"() -> (w541:string)
            n234 = global read "Global textParse.vi" "Speed Pot Voltage Tol. Max"() -> (w550:string)
            n235 = global read "Global textParse.vi" "Speed Pot Voltage Tol. Min"() -> (w553:string)
            n236 = global read "Global textParse.vi" "Speed Pot Voltage Tol. Min"() -> (w540:string)
            n237 = global read "Global textParse.vi" "Speed Pot Voltage Tol. Min"() -> (w549:string)
            n238 = call "Dual output square wave 180 out of phase.vi"("VISA resource name"=w559, "Enable Output 1"=TRUE, "error in (no error)"=w544) -> ("error out"=w545:errorcluster)  [unwired: 23 in, 1 out]
            n239 = call "Voltage tolerance.vi"("Data Sample"=80.0, "Spec Output"=w555, "Upper"=w554, "Lower"=w553) -> ("Boolean"=→"Boolean 2":bool)  [unwired: 10 in, 1 out]
            n240 = call "Voltage tolerance.vi"("Data Sample"=105.0, "Spec Output"=w542, "Upper"=w541, "Lower"=w540) -> ("Boolean"=→"Boolean 3":bool)  [unwired: 10 in, 1 out]
            n241 = call "Voltage tolerance.vi"("Data Sample"=130.0, "Spec Output"=w551, "Upper"=w550, "Lower"=w549) -> ("Boolean"=→"Boolean":bool)  [unwired: 10 in, 1 out]
            n242 = call "Sampled Data.vi"("Error In"=w545, "Data Sample"=23.0, "refnum in"=w578) -> ("refnum out"=w575:refnum<file>)  [unwired: 7 in, 1 out]
            n243 = call "Sampled Data.vi"("Data Sample"=123.0, "refnum in"=w575) -> ("error out"=w557:errorcluster, "refnum out"=w574:refnum<file>)  [unwired: 8 in]
            n244 = call "Sampled Data.vi"("Error In"=w557, "Data Sample"=34.0, "refnum in"=w574) -> ("error out"=w556:errorcluster, "refnum out"=w573:refnum<file>)  [unwired: 7 in]
            n245 = call "Sampled Data.vi"("Error In"=w556, "Data Sample"=765.0, "refnum in"=w573) -> ("refnum out"=w572:refnum<file>)  [unwired: 7 in, 1 out]
            n246 = call "Sampled Data.vi"("Data Sample"=234.0, "refnum in"=w572) -> ("refnum out"=w571:refnum<file>)  [unwired: 8 in, 1 out]
            n247 = call "Sampled Data.vi"("Data Sample"=4532.0, "refnum in"=w571) -> ("refnum out"=w570:refnum<file>)  [unwired: 8 in, 1 out]
            n248 = call "Sampled Data.vi"("Data Sample"=543.0, "refnum in"=w570) -> ("error out"=w543:errorcluster, "refnum out"=w569:refnum<file>)  [unwired: 8 in]
            n249 = Select(t=T3."Fail", s=w579, f=T3."Another") -> (s? t:f=w583:T3)
            n250 = Not(x=w579) -> (.not. x?=w581:bool)
            n251 = case shown="False" w581 {
              tunnel: w569 -> [w588 w591]
              tunnel: [w588 w592] -> w580
              tunnel: [w587 w589] -> w576
              tunnel: w543 -> [w587 _]
              frame False {
              }
              frame True {
                n252 = Write to Text File(file (use dialog)=w591, text="PASSED") -> (refnum out=w592:refnum<file>, error out=w589:errorcluster)  [unwired: 2 in, 1 out]
              }
            }
            n253 = call <vilib>:"Simple Error Handler.vi"("error in (no error)"=w576) -> ("error out"=w584:errorcluster)  [unwired: 4 in, 4 out]
          }
          frame 6 {
            # "Another"
            n254 = call "Prompt User for Input"() -> ("Yes"=w593:bool)  [unwired: 18 in, 1 out]
            n255 = Select(t=T3."SW Read", s=w593, f=T3."Close") -> (s? t:f=w597:T3)
            n256 = call <vilib>:"Simple Error Handler.vi"() -> ("error out"=w596:errorcluster)  [unwired: 5 in, 4 out]
          }
          frame 7 {
            # "Fail"
            n257 = call "Prompt User for Input2"() -> ("error out"=w600:errorcluster)  [unwired: 18 in, 1 out]
            n258 = Write to Text File(file (use dialog)=w602, text="FAILED") -> (refnum out=w603:refnum<file>)  [unwired: 2 in, 2 out]
            n259 = call <vilib>:"Simple Error Handler.vi"("error in (no error)"=w600) -> ("error?"=w604:bool, "error out"=w605:errorcluster)  [unwired: 4 in, 3 out]
          }
          frame 8 {
            # "extract file path and file name"
            # "Close"
            n260 = call "Close Data File and open.vi"("File Refnum In"=w619) -> ("error out"=w608:errorcluster, "path"=w618:path)  [unwired: 9 in]
            n261 = Path To String(path=w618) -> (string=w615:string)
            n262 = Reverse String(1:w615) -> (0:w614:string)
            n263 = Search/Split String(string=w615, offset (0)=113) -> (substring before match=w610:string)  [unwired: 1 in, 2 out]
            "File Path" <- w610
            n264 = Search/Split String(string=w614, offset (0)=32) -> (substring before match=w612:string)  [unwired: 1 in, 2 out]
            n265 = Reverse String(1:w612) -> (0:w613:string)
            n266 = Search/Split String(string=w613, offset (0)=28) -> (substring before match=w609:string)  [unwired: 1 in, 2 out]
            "File Name" <- w609
            n267 = call "CMD execution.vi"("Path"=w610, "File name"=w609, "error in (no error)"=w608) -> ("error out"=w607:errorcluster)  [unwired: 12 in]
            n268 = call <vilib>:"Simple Error Handler.vi"("error in (no error)"=w607) -> ("error out"=w621:errorcluster)  [unwired: 4 in, 4 out]
          }
        }
        n269 = Or(x=w12, y="E-STOP") -> (x .or. y?=w11:bool)
      }
    }
    frame "Instumentation Test" {
      n270 = call "Instrumentation Controls.vi"("VISA DS"=refnum<visa-resource-name> refnum, "VISA DM"=refnum<visa-resource-name> "USB0::0x1AB1::0x0C94::DM3O194400985::INSTR", "VISA DG"=refnum<visa-resource-name> "USB0::0x1AB1::0x0641::DG4E202501630::INSTR") -> ("DS"=→"DS":bool, "DM"=→"DM":bool, "DG"=→"DG":bool)  [unwired: 6 in]
    }
    frame "USB Scanner Setup" {
      w636 = ""
      n271 = property on="bar code" class="Str"("Key Focus"=TRUE) -> (error out=w637:errorcluster)  [unwired: 2 in, 1 out]
      n272 = local write "bar code"(w636) -> ()
      n273 = case shown="No Error" w637 {
        selector: w637 -> [w641 w648]
        tunnel: [w642 "Bad Scan" ("bar code")] -> w635
        tunnel: w636 -> [w640 _]
        tunnel: [w639 w648] -> w630
        frame No Error {
          n274 = while {
            tunnel: ["bar code"] -> w642
            tunnel: w641 -> [w643]
            tunnel: w640 -> [_]
            tunnel: [w643] -> w639
            stop <- "stop" stop-if-true
            n275 = Wait (ms)(milliseconds to wait=u32 100) -> ()  [unwired: 1 out]
          }
        }
        frame Error {
        }
      }
      "bar code read" <- w635
      n276 = call <vilib>:"Simple Error Handler.vi"("error in (no error)"=w630) -> ("error?"=→"error?":bool)  [unwired: 4 in, 4 out]
      n277 = Search/Split String(string=w635, offset (0)=6) -> (substring before match=w633:string)  [unwired: 1 in, 2 out]
      n278 = Concatenate Strings(w633, ".txt" ("string")) -> (→"concatenated string":string)
    }
    frame "Procedure" {
      n279 = case shown="1" "Documentation" {
        frame 0, Default {
          # "Displays Software Version"
          n280 = call-poly <vilib>:"Read Delimited Spreadsheet.vi"("file path (dialog if empty)"=path "C:/Users/bryan.lee/Desktop/Specification sheets/Documentation/...Software Version.txt") -> ("all rows"=→"SW Version":string[][])  [unwired: 9 in, 5 out]
        }
        frame 1 {
          # "Opens Procedure"
          n281 = while {
            i -> [w653]
            stop <- w652 stop-if-true
            n282 = call "CMD execution.vi"() -> ()  [unwired: 15 in, 1 out]
            n283 = Equal?(x=w653, y=u16 0) -> (x = y?=w652:bool)
          }
        }
        frame 2 {
          # "Opens Procedure"
          n284 = while {
            i -> [w657]
            stop <- w656 stop-if-true
            n285 = call "CMD execution.vi"("File name"="Equipment Verification") -> ()  [unwired: 14 in, 1 out]
            n286 = Equal?(x=w657, y=u16 0) -> (x = y?=w656:bool)
          }
        }
      }
    }
  }
